vi "Is Group Active.vi"(8 "error in (no error)":errorcluster, 10 "plugin iteration":u64=1, 11 "Transfer Group Timing in":refnum<class "Transfer Group Timing.lvclass">) -> (0 "error out":errorcluster, 2 "active?":bool, 3 "Transfer Group Timing out":refnum<class "Transfer Group Timing.lvclass">)   [LabVIEW 2017, in "DSF Core.lvlib" / "Transfer Group Timing.lvclass"]
uses:
  Transfer Group Timing.lvclass
  Transfer Group Timing.lvclass/Transfer Group Timing.ctl
  Timing.lvclass/Timing.ctl
  Get Decimation.vi
  Get Offset.vi
  Timing.lvclass
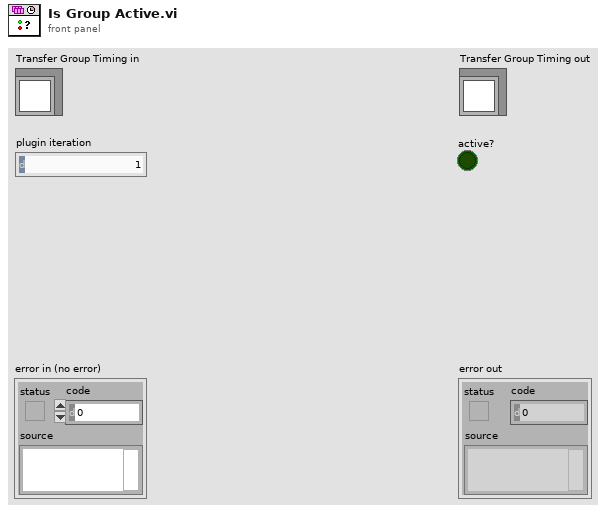
[diagram p1: front panel]
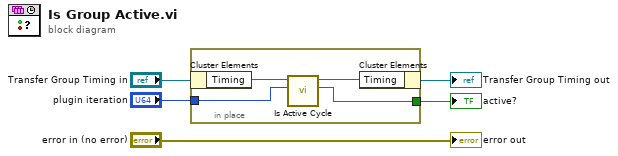
[diagram p0: block diagram]
diagram:
  n1 = in-place {
    in-place-border: "plugin iteration" -> [w7]
    in-place-border: [w6] -> w2
    n2 = in-place-cluster #1("Transfer Group Timing in") -> ("Timing"=w9:refnum<class "Timing.lvclass">)
    n3 = call "Is Active Cycle.vi"("iteration"=w7, "Timing in"=w9) -> ("active?"=w6:bool, "Timing out"=w8:refnum<class "Timing.lvclass">)  [unwired: 8 in]
    n4 = in-place-cluster #1("Timing"=w8) -> (→"Transfer Group Timing out":refnum<class "Transfer Group Timing.lvclass">)
  }
  "active?" <- w2
  "error out" <- "error in (no error)"
